vi "find_max_min_freq_in_spectra_cluster.vi"(4 "Array":T1(array[cluster]), 5 "freq offset":dbl) -> (0 "min freq":dbl, 2 "max freq":dbl)   [LabVIEW 2011]
doc: "Takes an array of spectra cluster and calculates the highest and lowest frequency."
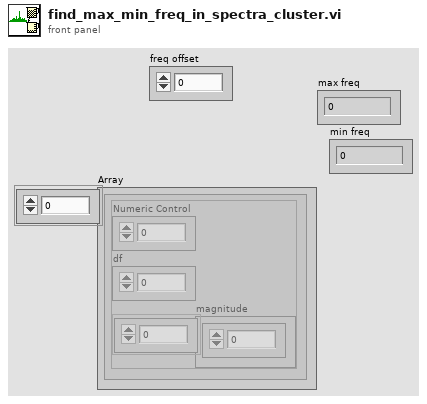
[diagram p1: front panel]
types:
  T1 = cluster{"Numeric Control":dbl, "df":dbl, "magnitude":dbl[]}[]
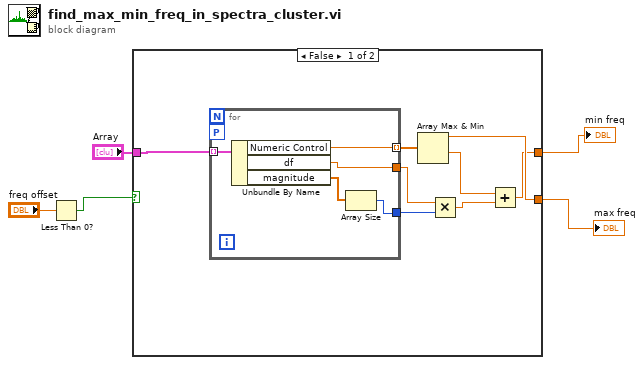
[diagram p0: block diagram]
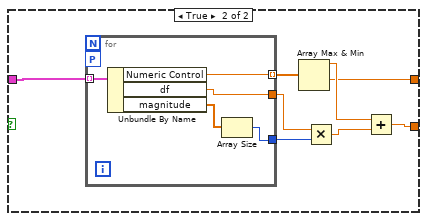
[diagram p2: hidden frame]
diagram:
  n1 = Less Than 0?(x="freq offset") -> (x < 0?=w3:bool)
  n2 = case shown="False" w3 {
    tunnel: "Array" -> [w8 w22]
    tunnel: [w7 w20] -> w5
    tunnel: [w6 w19] -> w2
    frame False {
      n3 = for {
        tunnel: w8 -> [w18] mode=indexing
        tunnel: [w17] -> w13 mode=indexing
        tunnel: [w15] -> w12
        tunnel: [w14] -> w11
        workers-P: _ -> [_]
        n4 = Unbundle By Name(w18) -> ("Numeric Control"=w17:dbl, "df"=w15:dbl, "magnitude"=w16:dbl[])
        n5 = Array Size(array=w16) -> (size(s)=w14:i32)
      }
      n6 = Array Max & Min(array=w13) -> (max value=w7:dbl, min value=w10:dbl)  [unwired: 2 out]
      n7 = Multiply(x=w12, y=w11) -> (x*y=w9:dbl)
      n8 = Add(x=w10, y=w9) -> (x+y=w6:dbl)
    }
    frame True {
      n9 = for {
        tunnel: w22 -> [w31] mode=indexing
        tunnel: [w30] -> w26 mode=indexing
        tunnel: [w28] -> w25
        tunnel: [w27] -> w24
        workers-P: _ -> [_]
        n10 = Unbundle By Name(w31) -> ("Numeric Control"=w30:dbl, "df"=w28:dbl, "magnitude"=w29:dbl[])
        n11 = Array Size(array=w29) -> (size(s)=w27:i32)
      }
      n12 = Array Max & Min(array=w26) -> (max value=w21:dbl, min value=w19:dbl)  [unwired: 2 out]
      n13 = Multiply(x=w25, y=w24) -> (x*y=w23:dbl)
      n14 = Add(x=w21, y=w23) -> (x+y=w20:dbl)
    }
  }
  "max freq" <- w5
  "min freq" <- w2
